vi "HB_Simple.Main Very Simple.vi"() -> ()   [LabVIEW 2009, in "HB_BaseClass_Examples.lvlib"]
doc: "Simple demo VI."
uses:
  HB_BaseClass_Examples.lvlib
  HB_Simple.lvclass
  lib.lib/HGF_LVC/HGF_Auxiliary/HGF_Auxiliary.lvlib
panel:
  out "x 2":dbl
  out "x 1":dbl
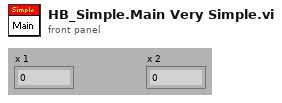
[diagram p1: front panel]
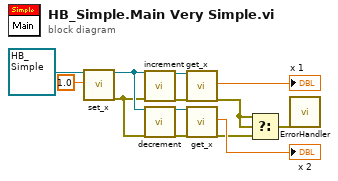
[diagram p0: block diagram]
diagram:
  n1 = call "set_x.vi"("HB_Simple"=refnum<class "HB_Simple.lvclass"> refnum ("HGF_BaseClass_Examples.lvlib:HB_Simple.lvclass"), "x"=1.0) -> ("dup HB_Simple"=w2:refnum<class "HB_Simple.lvclass">, "error out"=w1:errorcluster)  [unwired: 1 in, 15 out]
  n2 = call "increment.vi"("HB_Simple in"=w2, "error in (no error)"=w1) -> ("HB_Simple out"=w13:refnum<class "HB_Simple.lvclass">, "error out"=w8:errorcluster)  [unwired: 16 in]
  n3 = call "decrement.vi"("HB_Simple in"=w2, "error in (no error)"=w1) -> ("HB_Simple out"=w3:refnum<class "HB_Simple.lvclass">, "error out"=w7:errorcluster)  [unwired: 16 in]
  n4 = call "get_x.vi"("HB_Simple"=w13, "error in (no error)"=w8) -> ("x"=→"x 1":dbl, "error out"=w6:errorcluster)  [unwired: 16 out]
  n5 = call "get_x.vi"("HB_Simple"=w3, "error in (no error)"=w7) -> ("x"=→"x 2":dbl, "error out"=w5:errorcluster)  [unwired: 16 out]
  n6 = Select(t=w6, s=w6, f=w5) -> (s? t:f=w4:errorcluster)
  n7 = call "ErrorHandler.vi"("error in (no error)"=w4) -> ()  [unwired: 6 in, 13 out]
